vi "test-PID-input-output.vi"() -> ()   [LabVIEW 2019]
uses:
  <vilib>/Rock Robotics/WPI/ThirdParty/JAS_Junk/TrajLib/PIDController_NewPeriod.vi
  <vilib>/Rock Robotics/WPI/ThirdParty/JAS_Junk/TrajLib/PIDController_SetSetpoint.vi
  <vilib>/Rock Robotics/WPI/ThirdParty/JAS_Junk/TrajLib/PIDController_Calculate_PV.vi
  <vilib>/Rock Robotics/SystemInterfaces/NetworkCommunication/NetComm_UsageReport_report.vi
  <vilib>/Rock Robotics/WPI/ThirdParty/JAS_Junk/TrajLib/ControllerUtil_GetModulusError.vi
  <vilib>/Rock Robotics/WPI/ThirdParty/JAS_Junk/TrajLib/Util_LibraryGlobals.vi
  <vilib>/Rock Robotics/WPI/ThirdParty/JAS_Junk/TrajLib/Trajectory_Library.lvlib
  <vilib>/Rock Robotics/WPI/ThirdParty/JAS_Junk/TrajLib/PID_CONTROLLER.ctl
panel:
  out "T0 PID CTRL":T1={"Kp"=0.0, "Ki"=0.0, "Kd"=0.0, "Period"=0.0, "Max_Integral"=0.0, "Min_Integral"=0.0, "Max_Input"=0.0, "Min_Input"=0.0, "Continuous"=FALSE, "PositionError"=0.0, "VelocityError"=0.0, "PrevError"=0.0, "TotalError"=0.0, "PositionTolerance"=0.0, "VelocityTolerance"=0.0, "SetPoint"=0.0, "Kf"=0.0, "Prev_Deriv"=0.0, "Prev_Deriv 2"=0.0, "DerivativeFilter"=FALSE, "Min_Output"=-9.99e+35, "Max_Output"=9.9e+35, "Prev_F_P"=0.0, "Prev_F_P_2"=0.0, "AntiWindupActive"=FALSE, "Measurement"=0.0} {"Measurement" format="%16_6e"; "Prev_F_P_2" format="%16_6e"; "Prev_F_P" format="%16_6e"; "Max_Output" format="%16_6e"; "Min_Output" format="%16_6e"; "Prev_Deriv 2" format="%16_6e"; "Prev_Deriv" format="%16_6e"; "Kf" format="%16_6e"; "SetPoint" format="%16_6e"; "VelocityTolerance" format="%16_6e"; "PositionTolerance" format="%16_6e"; "TotalError" format="%16_6e"; "PrevError" format="%16_6e"; "VelocityError" format="%16_6e"; "PositionError" format="%16_6e"; "Min_Input" format="%16_6e"; "Max_Input" format="%16_6e"; "Min_Integral" format="%16_6e"; "Max_Integral" format="%16_6e"; "Period" format="%16_6e"; "Kd" format="%16_6e"; "Ki" format="%16_6e"; "Kp" format="%16_6e"}
  out "T3 -- Output =":dbl
  out "T2 -- Output  = -0.01":dbl
  out "T1 -- Output  = -0.1":dbl
  out "T0 -- Output < 0":dbl
  # "PID Input Output"
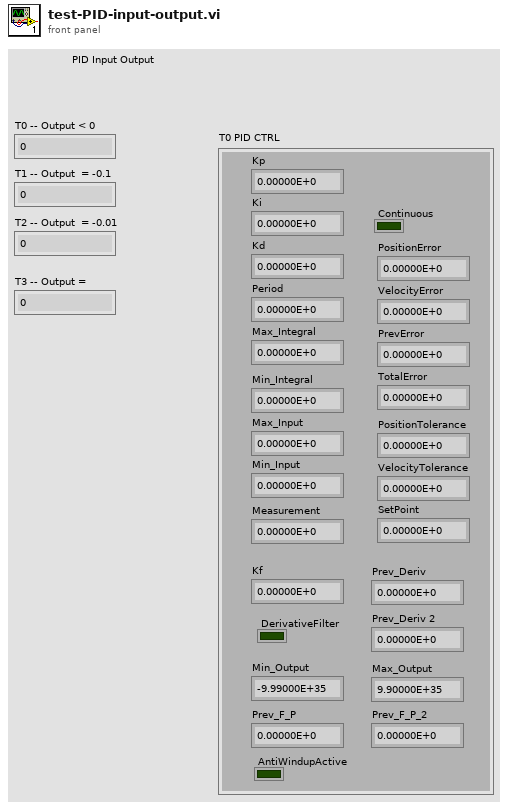
[diagram p1: front panel]
types:
  T1 = typedef "Trajectory_Library.lvlib/PID_CONTROLLER.ctl" = cluster{"Kp":dbl, "Ki":dbl, "Kd":dbl, "Period":dbl, "Max_Integral":dbl, "Min_Integral":dbl, "Max_Input":dbl, "Min_Input":dbl, "Continuous":bool, "PositionError":dbl, "VelocityError":dbl, "PrevError":dbl, "TotalError":dbl, "PositionTolerance":dbl, "VelocityTolerance":dbl, "SetPoint":dbl, "Kf":dbl, "Prev_Deriv":dbl, "Prev_Deriv 2":dbl, "DerivativeFilter":bool, "Min_Output":dbl, "Max_Output":dbl, "Prev_F_P":dbl, "Prev_F_P_2":dbl, "AntiWindupActive":bool, "Measurement":dbl}
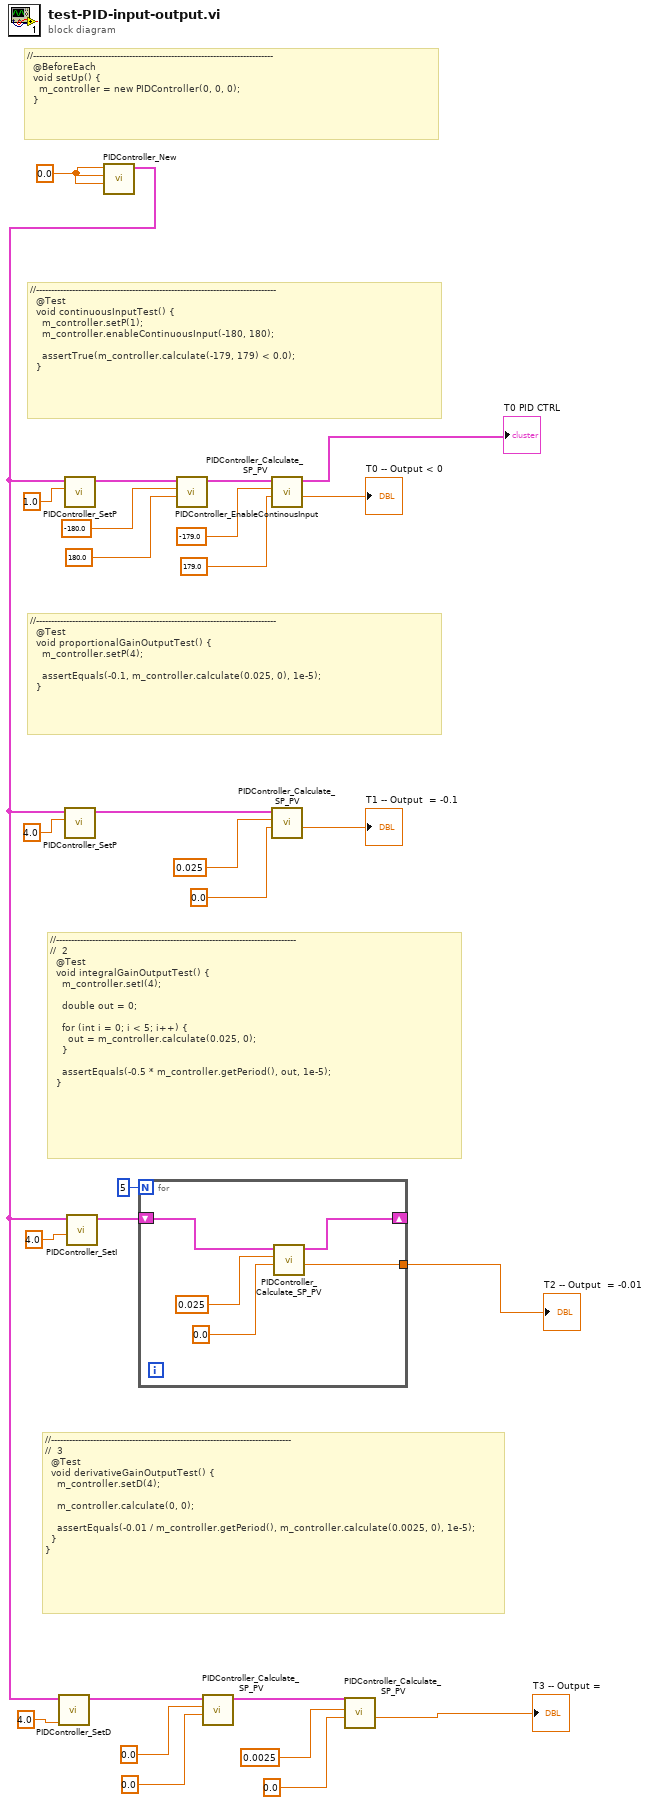
[diagram p0: block diagram]
diagram:
  w28 = 0.0 ("Kp")
  # "//--------------------------------------------------------------------------------\n//  3\n  @Test\n  void derivativeGainOutputTest() {\n    m_controller.setD(4);\n\n    m_controller.calculate(0, 0);\n\n    assertEquals(-0.01 / m_controller.getPeriod(), m_controller.calculate(0.0025, 0), 1e-5);\n  }\n}"
  # "//--------------------------------------------------------------------------------\n//  2\n  @Test\n  void integralGainOutputTest() {\n    m_controller.setI(4);\n\n    double out = 0;\n\n    for (int i = 0; i < 5; i++) {\n      out = m_controller.calculate(0.025, 0);\n    }\n\n    assertEquals(-0.5 * m_controller.getPeriod(), out, 1e-5);\n  }"
  # "//--------------------------------------------------------------------------------\n  @Test\n  void proportionalGainOutputTest() {\n    m_controller.setP(4);\n\n    assertEquals(-0.1, m_controller.calculate(0.025, 0), 1e-5);\n  }"
  # "//--------------------------------------------------------------------------------\n  @BeforeEach\n  void setUp() {\n    m_controller = new PIDController(0, 0, 0);\n  }"
  # "//--------------------------------------------------------------------------------\n  @Test\n  void continuousInputTest() {\n    m_controller.setP(1);\n    m_controller.enableContinuousInput(-180, 180);\n\n    assertTrue(m_controller.calculate(-179, 179) < 0.0);\n  }"
  n1 = call <vilib>:"PIDController_New.vi"("Kd"=w28, "Ki"=w28, "Kp"=w28) -> ("PID_CONTROLLER"=w6:T1)  [unwired: 8 in]
  n2 = call <vilib>:"PIDController_SetD.vi"("Kd"=4.0 ("Kp"), "in PID_CONTROLLER"=w6) -> ("out PID_CONTROLLER"=w9:T1)  [unwired: 9 in]
  n3 = call <vilib>:"PIDController_SetP.vi"("Kp"=1.0, "in PID_CONTROLLER"=w6) -> ("out PID_CONTROLLER"=w26:T1)  [unwired: 9 in]
  n4 = call <vilib>:"PIDController_SetP.vi"("Kp"=4.0, "in PID_CONTROLLER"=w6) -> ("out PID_CONTROLLER"=w15:T1)  [unwired: 9 in]
  n5 = call <vilib>:"PIDController_SetI.vi"("Ki"=4.0 ("Kp"), "in PID_CONTROLLER"=w6) -> ("out PID_CONTROLLER"=w12:T1)  [unwired: 9 in]
  n6 = for {
    N: 5 -> [_]
    tunnel: [w31] -> w13
    shift-right: [w29] -> _
    shift-left: w12 -> [w30]
    n7 = call <vilib>:"PIDController_Calculate_SP_PV.vi"("SP-SetPoint"=0.0, "PV-Measurement"=0.025, "in PID_CONTROLLER"=w30) -> ("CO-ControlOutput"=w31:dbl, "out PID_CONTROLLER"=w29:T1)  [unwired: 7 in]
  }
  "T2 -- Output  = -0.01" <- w13
  n8 = call <vilib>:"PIDController_EnableContinousInput.vi"("MaxInput"=180.0, "MinInput"=-180.0, "in PID_CONTROLLER"=w26) -> ("out PID_CONTROLLER"=w23:T1)  [unwired: 8 in]
  n9 = call <vilib>:"PIDController_Calculate_SP_PV.vi"("SP-SetPoint"=0.0, "PV-Measurement"=0.0, "in PID_CONTROLLER"=w9) -> ("out PID_CONTROLLER"=w3:T1)  [unwired: 7 in, 1 out]
  n10 = call <vilib>:"PIDController_Calculate_SP_PV.vi"("SP-SetPoint"=179.0, "PV-Measurement"=-179.0, "in PID_CONTROLLER"=w23) -> ("CO-ControlOutput"=→"T0 -- Output < 0":dbl, "out PID_CONTROLLER"=→"T0 PID CTRL":T1)  [unwired: 7 in]
  n11 = call <vilib>:"PIDController_Calculate_SP_PV.vi"("SP-SetPoint"=0.0, "PV-Measurement"=0.025, "in PID_CONTROLLER"=w15) -> ("CO-ControlOutput"=→"T1 -- Output  = -0.1":dbl)  [unwired: 7 in, 1 out]
  n12 = call <vilib>:"PIDController_Calculate_SP_PV.vi"("SP-SetPoint"=0.0, "PV-Measurement"=0.0025, "in PID_CONTROLLER"=w3) -> ("CO-ControlOutput"=→"T3 -- Output =":dbl)  [unwired: 7 in, 1 out]
